vi "_RT_CtrlLoop_Log packageMessage.vi"(0 "logCluster":T1) -> (1 "igore":bool, 2 "Message":string)   [LabVIEW 2018]
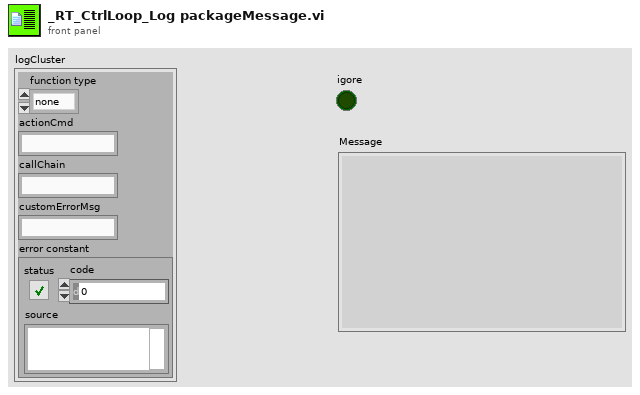
[diagram p1: front panel]
types:
  T1 = cluster{"function type":enum16{"none", "init", "write", "read"}, "actionCmd":string, "callChain":string, "customErrorMsg":string, "error constant":errorcluster}
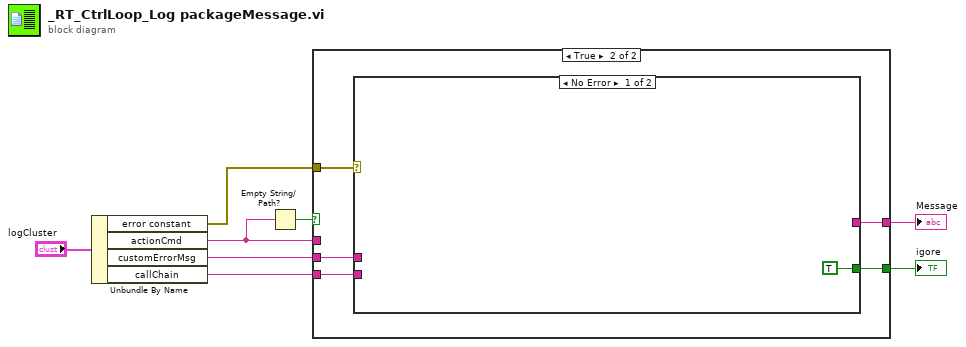
[diagram p0: block diagram]
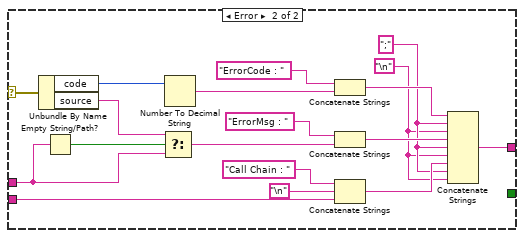
[diagram p3: hidden frame]
diagram:
  n1 = Unbundle By Name("logCluster") -> ("error constant"=w2:errorcluster, "actionCmd"=w6:string, "customErrorMsg"=w5:string, "callChain"=w4:string)
  n2 = Empty String/Path?(string/path=w6) -> (empty?=w7:bool)
  n3 = case shown="True" w7 {
    tunnel: w6 -> [w9 _]
    tunnel: [w9 w10] -> w1
    tunnel: w5 -> [_ w13]
    tunnel: w4 -> [_ w12]
    tunnel: [_ w14] -> w3
    tunnel: w2 -> [_ w11]
    frame False {
    }
    frame True {
      n4 = case shown="No Error" w11 {
        selector: w11 -> [_ w25]
        tunnel: [TRUE _] -> w14
        tunnel: w13 -> [_ w32]
        tunnel: w12 -> [_ w22]
        tunnel: [_ w16] -> w10
        frame No Error {
        }
        frame Error {
          w18 = ";" ("string")
          w17 = "\n"
          n5 = Unbundle By Name(w25) -> ("code"=w31:i32, "source"=w24:string)
          n6 = Empty String/Path?(string/path=w32) -> (empty?=w33:bool)
          n7 = Select(t=w24, s=w33, f=w32) -> (s? t:f=w23:string)
          n8 = Number To Decimal String(number=w31) -> (decimal integer string=w26:string)  [unwired: 1 in]
          n9 = Concatenate Strings("ErrorCode : " ("string"), w26) -> (w21:string)
          n10 = Concatenate Strings("ErrorMsg : " ("string"), w23) -> (w20:string)
          n11 = Concatenate Strings("Call Chain : " ("string"), "\n", w22) -> (w19:string)
          n12 = Concatenate Strings(w21, w18, w17, w20, w18, w17, w19, w18, w17) -> (w16:string)
        }
      }
    }
  }
  "Message" <- w1
  "igore" <- w3
